vi "intCSMs.vi"(8 "error in (no error)":errorcluster, 11 "TestCase in":refnum<class "testcase-CSMSubModule.lvclass">) -> (0 "error out":errorcluster, 3 "TestCase out":refnum<class "testcase-CSMSubModule.lvclass">)   [LabVIEW 2017, in "testcase-CSMSubModule.lvclass"]
uses:
  testcase-CSMSubModule.lvclass
  testcase-CSMSubModule.lvclass/testcase-CSMSubModule.ctl
  CSM/Normal-CSM.vi
  CSM/CSM-Testcase.lvlib
  src/user.lib/_NEVSTOP/Communicable State Machine(CSM)/Communicable State Machine.lvlib
panel:
  out "CSMs Left":string[](array[string])
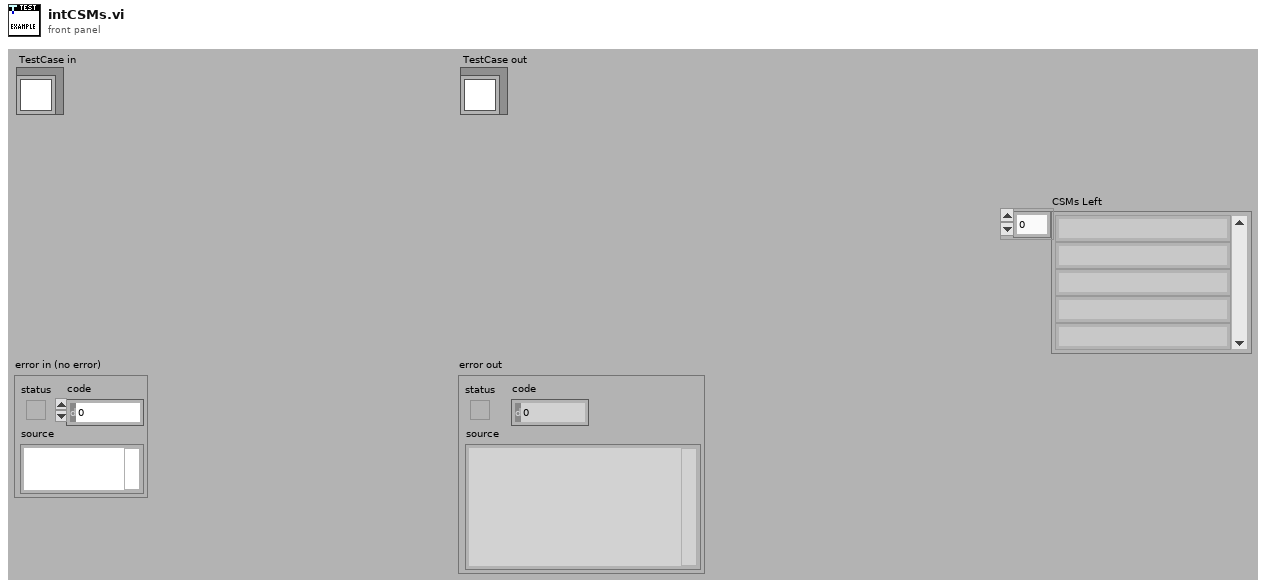
[diagram p1: front panel]
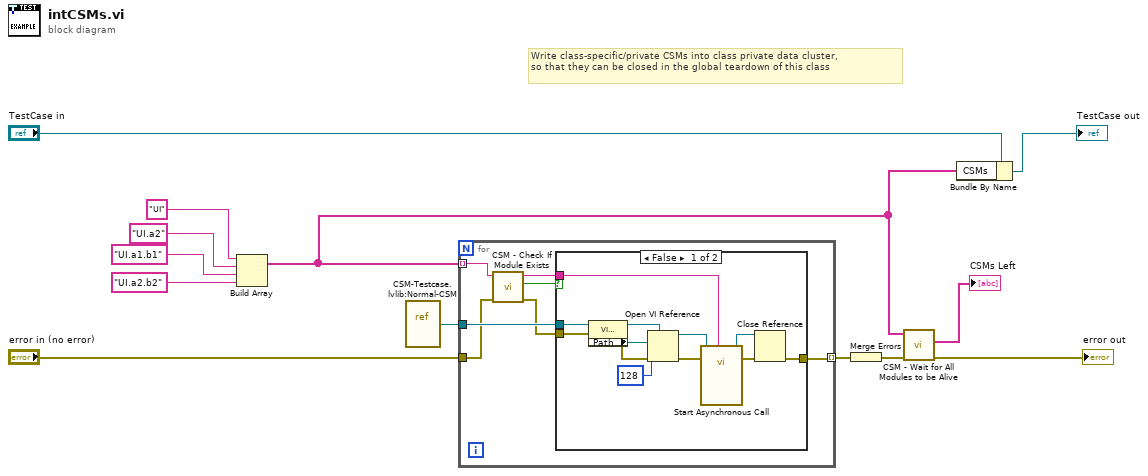
[diagram p0: block diagram]
diagram:
  # "Write class-specific/private CSMs into class private data cluster,\nso that they can be closed in the global teardown of this class"
  n1 = Build Array("UI" ("Name (\"\" to Use UUID)"), "UI.a2" ("Name (\"\" to Use UUID)"), "UI.a1.b1" ("Name (\"\" to Use UUID)"), "UI.a2.b2" ("Name (\"\" to Use UUID)")) -> (w5:string[])
  n2 = vi-ref "CSM-Testcase.lvlib:Normal-CSM.vi"() -> (w11:refnum<vi>)
  n3 = for {
    tunnel: w11 -> [w20]
    tunnel: w5 -> [w17] mode=indexing
    tunnel: "error in (no error)" -> [w19]
    tunnel: [w14] -> w2 mode=indexing
    n4 = call "CSM - Check If Module Exists.vi"("Error In"=w19, "CSM Name"=w17) -> ("error out"=w18:errorcluster, "Exist?"=w15:bool, "CSM Name (Dup)"=w16:string)  [unwired: 7 in]
    n5 = case shown="False" w15 {
      tunnel: w20 -> [w24 _]
      tunnel: [w23 w33] -> w14
      tunnel: w18 -> [w22 w33]
      tunnel: w16 -> [w21 _]
      frame False {
        n6 = property class="VI (strict)"(reference=w24, error in=w22) -> (reference out=w30:refnum<vi>, error out=w28:errorcluster, "Path"=w27:path)
        n7 = Open VI Reference(type specifier VI Refnum (for type only)=w30, vi path=w27, options=128, error in (no error)=w28) -> (vi reference=w26:refnum<vi>, error out=w31:errorcluster)  [unwired: 2 in]
        n8 = call-by-ref "Start Asynchronous Call"(reference=w26, error in=w31, "Name (\"\" to Use UUID)"=w21) -> (reference out=w25:refnum<vi>, error out=w29:errorcluster)  [unwired: 11 in]
        n9 = Close Reference(reference=w25, error in (no error)=w29) -> (error out=w23:errorcluster)
      }
      frame True {
      }
    }
  }
  n10 = Merge Errors(w2) -> (w1:errorcluster)
  n11 = call "CSM - Wait for All Modules to be Alive.vi"("Error In"=w1, "CSM Names"=w5) -> ("error out"=→"error out":errorcluster, "CSMs Left"=→"CSMs Left":string[])  [unwired: 7 in, 1 out]
  n12 = Bundle By Name(cluster="TestCase in", "CSMs"=w5) -> (→"TestCase out":refnum<class "testcase-CSMSubModule.lvclass">)
